vi "Name.vi"(11 "Boolean Data Type in":refnum<class "Boolean Data Type.lvclass">) -> (2 "String":string="Generic", 3 "Boolean Data Type (dup)":refnum<class "Boolean Data Type.lvclass">)   [LabVIEW 2018, in "Boolean Data Type.lvclass"]
uses:
  Boolean Data Type.lvclass
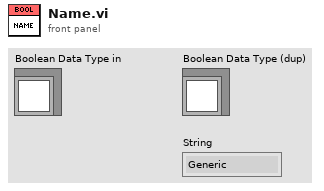
[diagram p1: front panel]
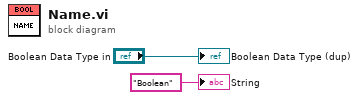
[diagram p0: block diagram]
diagram:
  "Boolean Data Type (dup)" <- "Boolean Data Type in"
  "String" <- "Boolean" ("String")
